vi "onStarted.vi"(8 "error in (no error)":errorcluster, 11 "system":refnum<class "multichannel-lockin.lvclass">) -> (0 "error out":errorcluster, 3 "system out":refnum<class "multichannel-lockin.lvclass">)   [LabVIEW 2019, in "multichannel-lockin.lvclass"]
doc: "JKI State Machine Objects (SMO) 1.2.1.55\nJKI - JKI\nCopyright (c) 2017, JKI"
uses:
  multichannel-lockin.lvclass
  C:/Program Files (x86)/National Instruments/LabVIEW 2019/vi.lib/JKI/JKI SMO/SMO/SMO.lvclass
  multichannel-lockin.lvclass/multichannel-lockin.ctl
  <userlib>/LevyLab/Instrument Framework/SMOs/Instrument/Instrument.lvclass
  DAQ_Manager/DAQ_Manager.lvclass
  DSP/DSP.lvclass
  Generator/Generator.lvclass
  Scope/Scope.lvclass
  <vilib>/JKI/JKI SMO/SMO/SMO.lvclass
panel:
  # "For instructions on how to use the JKI State Machine Objects, examples and video tutorials, visit:\nhttp://jki.net/state-machine-objects/\n\nJKI State Machine Objects™\nhttp://jki.net/state-machine-objects/\nCopyright (C) 2005-2015, JKI <info@jki.net>\nALL RIGHTS RESERVED"
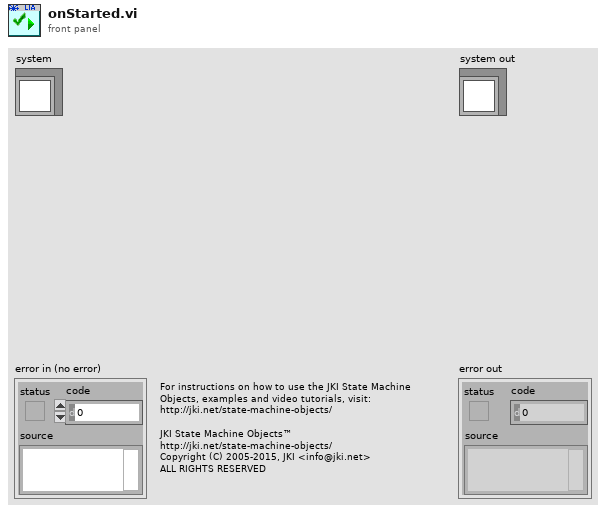
[diagram p1: front panel]
types:
  T1 = typedef "multichannel-lockin.lvclass/Dependencies-cluster.ctl" = cluster{"DAQ_Manager":refnum<class "DAQ_Manager.lvclass">, "DSP":refnum<class "DSP.lvclass">, "Generator":refnum<class "Generator.lvclass">, "Scope":refnum<class "Scope.lvclass">}
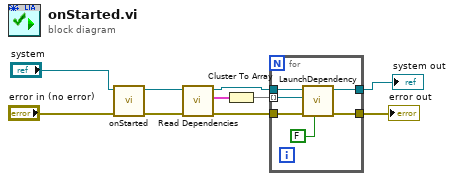
[diagram p0: block diagram]
diagram:
  n1 = call-parent "onStarted.vi"("error in (no error)"="error in (no error)", "SMO"="system") -> ("error out"=w4:errorcluster, "SMO out"=w7:refnum<class "multichannel-lockin.lvclass">)  [unwired: 8 in]
  n2 = call "Read Dependencies.vi"("error in (no error)"=w4, "system in"=w7) -> ("error out"=w3:errorcluster, "Dependencies"=w6:T1, "system"=w2:refnum<class "multichannel-lockin.lvclass">)  [unwired: 7 in]
  n3 = Cluster To Array(cluster=w6) -> (array=w5:refnum<class "SMO.lvclass">[])
  n4 = for {
    tunnel: w5 -> [w13] mode=indexing
    tunnel: w2 -> [w14]
    tunnel: w3 -> [w16]
    tunnel: [w15] -> w8
    tunnel: [w11] -> w1
    n5 = call <vilib>:"LaunchDependency.vi"("Shared Resource"=FALSE, "error in (no error)"=w16, "Dependency Type"=w13, "SMO in"=w14) -> ("error out"=w15:errorcluster, "SMO out"=w11:refnum<class "multichannel-lockin.lvclass">)  [unwired: 4 in, 2 out]
  }
  "error out" <- w8
  "system out" <- w1
